vi "NextState.vi"(0 "object in":refnum<class "SupportAttackerRole.lvclass">, 2 "Robot in":refnum<class "Robot.lvclass">, 4 "GameRef":refnum<data-value>, 5 "error in (no error)":errorcluster) -> (14 "object out":refnum<class "SupportAttackerRole.lvclass">, 16 "Robot out":refnum<class "Robot.lvclass">, 19 "error out":errorcluster)   [LabVIEW 2023, in "SupportAttackerRole.lvclass"]
uses:
  SupportAttackerRole.lvclass
  C:/Users/ebert/Documents/codes/SSL/repo/SSL_AI/NewSTP/NewRoles/Role_v2_class/Role_v2.lvclass
  Robot_class/Robot.lvclass
  Game_class/Game.lvclass
  SupportAttackerRole_states.ctl
  Robot_class/tactics.ctl
  Robot_class/Robot.lvclass/Robot.ctl
  Robot_class/Write tactic.vi
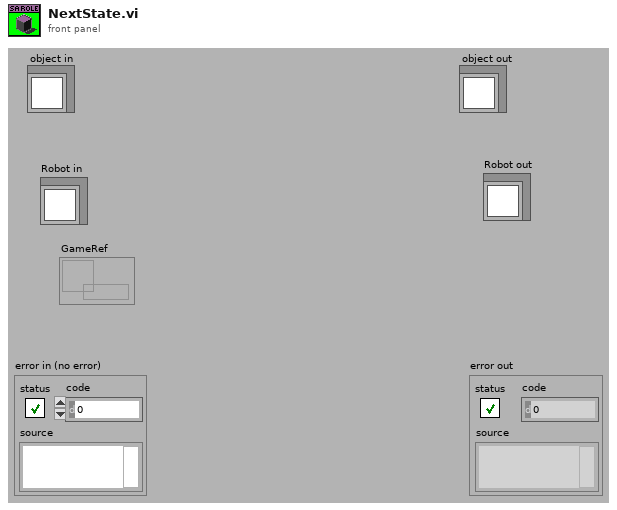
[diagram p1: front panel]
types:
  T1 = typedef "tactics.ctl" = enum16{"GoToBallPlacementPosition", "PlaceBall", "GoToBallPlacement", "5Robots", "BallPlacementEnemy", "ReceivePassInFuturePoint", "Roller", "PrepareRollToPassRollerGoTo", "PrepareRollToPassReceiverGoTo", "WaitRoll", "PositionToRoll", "PenaltyAttacker", "PassObserver", "PenaltyDefense", "TableReceiverTactic", "Test", "DefendGoal", "Marker", "FollowAttacker", "DefendArea", "Shoot", "AttackerAimGoal", "AttackerBallOutOfField", "AttackerBlock", "AttackerStop", "Duelist", "Halt", "ZigZag", "GoTo", "Timeout", "KickToBestRobot", "KickToPassReceiver", "PositionToReceivePass", "WaitPass", "Position", "Intercept", "PrepareShot", "Pass"}
  T2 = typedef "SupportAttackerRole.lvclass/SupportAttackerRole_states.ctl" = enum16{"Position", "WaitPass", "Exit"}
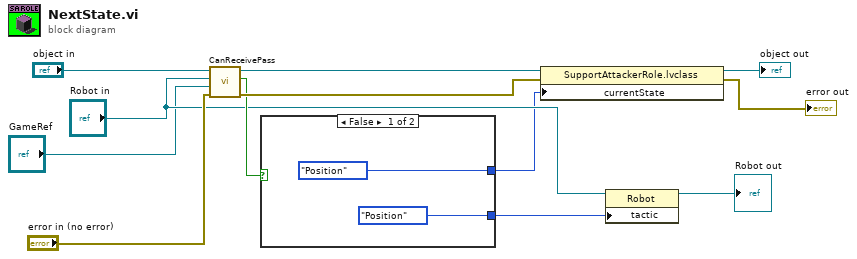
[diagram p0: block diagram]
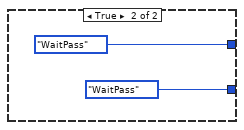
[diagram p2: hidden frame]
diagram:
  n1 = call-dynamic "CanReceivePass.vi"("error in (no error)"="error in (no error)", "GameRef"="GameRef", "Robot"="Robot in", "object in"="object in") -> ("error out"=w8:errorcluster, "CanReceivePass"=w6:bool, "object out"=w10:refnum<class "SupportAttackerRole.lvclass">)  [unwired: 5 in]
  n2 = case shown="False" w6 {
    tunnel: [tactics."Position" ("tactic") tactics."WaitPass" ("tactic")] -> w2
    tunnel: [SupportAttackerRole_states."Position" ("States") SupportAttackerRole_states."WaitPass" ("States")] -> w1
    frame False {
    }
    frame True {
    }
  }
  n3 = property class="SupportAttackerRole.lvclass"(reference=w10, error in=w8, "currentState"=w1) -> (reference out=→"object out":refnum<class "SupportAttackerRole.lvclass">, error out=→"error out":errorcluster)
  n4 = property class="Robot"(reference="Robot in", "tactic"=w2) -> (reference out=→"Robot out":refnum<class "Robot.lvclass">)  [unwired: 1 in, 1 out]
